vi "GetUserName.vi"() -> (0 "UserName":string)   [LabVIEW 2011]
uses:
  Advapi32.dll
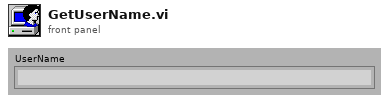
[diagram p1: front panel]
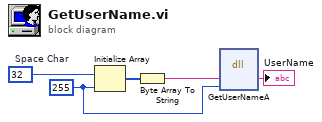
[diagram p0: block diagram]
diagram:
  w2 = 255 ("dimension size")
  w5 = u8 32  # Space Char
  n1 = Initialize Array(w5, w2) -> (w4:u8[])
  n2 = Byte Array To String(unsigned byte array=w4) -> (string=w3:string)
  n3 = dll-call lib="advapi32.dll" fn="GetUserNameA"("lpBuffer"=w3, "nSize"=w2) -> ("lpBuffer"=→"UserName":string)  [unwired: 3 in, 4 out]
